vi "Get SMO Public API.vi"(8 "error in (no error)":errorcluster, 11 "instrument.OptiCool in":refnum<class "instrument.OptiCool.lvclass">) -> (0 "error out":errorcluster, 2 "Commands":string[](array[string]), 3 "instrument.OptiCool out":refnum<class "instrument.OptiCool.lvclass">)   [LabVIEW 2019, in "instrument.OptiCool.lvclass"]
uses:
  instrument.OptiCool.lvclass
  <userlib>/_OpenG.lib/array/array.llb/Delete Elements from 1D Array (String)__ogtk.vi
  instrument.PPMS/instrument.PPMS.lvclass
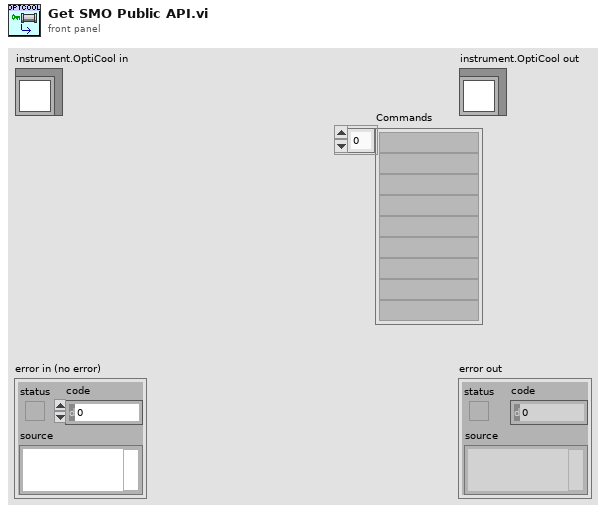
[diagram p1: front panel]
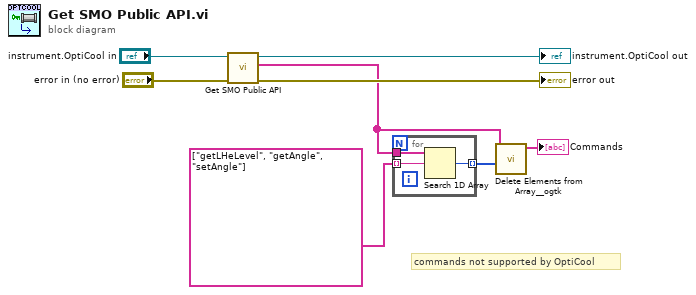
[diagram p0: block diagram]
diagram:
  # "commands not supported by OptiCool"
  n1 = call-parent "Get SMO Public API.vi"("error in (no error)"="error in (no error)", "instrument.PPMS in"="instrument.OptiCool in") -> ("error out"=→"error out":errorcluster, "Commands"=w2:string[], "instrument.PPMS out"=→"instrument.OptiCool out":refnum<class "instrument.OptiCool.lvclass">)  [unwired: 7 in]
  n2 = for {
    tunnel: [w11] -> w4 mode=indexing
    tunnel: string[] ["getLHeLevel", "getAngle", "setAngle"] ("Commands 2") -> [w10] mode=indexing
    tunnel: w2 -> [w9]
    n3 = Search 1D Array(1D array=w9, element=w10) -> (index of element=w11:i32)  [unwired: 1 in]
  }
  n4 = call-poly <userlib>:"Delete Elements from Array__ogtk.vi"("indices"=w4, "array"=w2) -> ("array w/ subset deleted"=→"Commands":string[])  [unwired: 8 in, 1 out]
